vi "1B.1-Spoof Centripital Acceleration.vi"(2 "Old Velocity":dbl[](array[numeric]), 3 "Rudder Angle":dbl) -> (0 "Speed":dbl, 1 "New Velocity":dbl[](array[numeric]))   [LabVIEW 2011]
doc: "This vi follows the formula A=([V_old,0]x[0,0,tan(Ra)/.3*norm(V_old)]);\nVnew=norm(V_old)/norm(V_old+A)*(V_old+A)\nThe magic number .3 indicated .3 meters between the rudder and the center of rotation"
uses:
  <vilib>/Analysis/_algsub.llb/Real Vector Norm.vi
  <vilib>/Analysis/NI_AALPro.lvlib
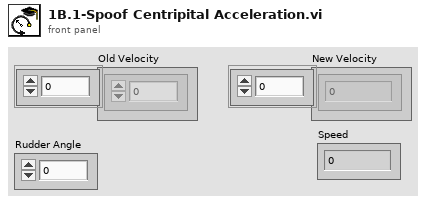
[diagram p1: front panel]
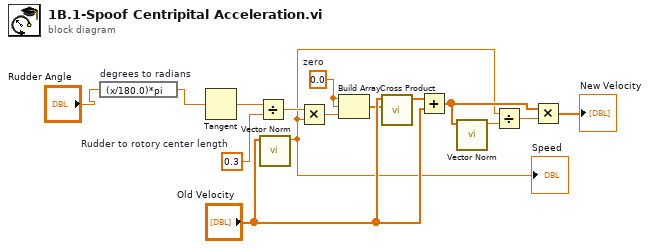
[diagram p0: block diagram]
diagram:
  w11 = 0.0  # zero
  w9 = 0.3  # Rudder to rotory center length
  n1 = expression code="(x/180.0)*pi" "degrees to radians"("Rudder Angle") -> (w1:dbl)
  n2 = Tangent(1:w1) -> (0:w8:dbl)
  n3 = Divide(x=w8, y=w9) -> (x/y=w10:dbl)
  n4 = call-poly <vilib>:"Vector Norm.vi"("Input Vector"="Old Velocity") -> ("norm"=w3:dbl)  [unwired: 9 in, 1 out]
  "Speed" <- w3
  n5 = Multiply(x=w10, y=w3) -> (x*y=w12:dbl)
  n6 = Build Array(w11, w11, w12) -> (w13:dbl[])
  n7 = call <vilib>:"Cross Product.vi"("B Vector"=w13, "A Vector"="Old Velocity") -> ("Cross Product"=w14:dbl[])  [unwired: 8 in, 1 out]
  n8 = Add(x=w14, y="Old Velocity") -> (x+y=w7:dbl[])
  n9 = call-poly <vilib>:"Vector Norm.vi"("Input Vector"=w7) -> ("norm"=w5:dbl)  [unwired: 9 in, 1 out]
  n10 = Divide(x=w3, y=w5) -> (x/y=w4:dbl)
  n11 = Multiply(x=w7, y=w4) -> (x*y=→"New Velocity":dbl[])
